vi "Sliding Menu Facade.vi"(0 "Data In":T5, 2 "Display State In":T2={"Numeric"=0.0, "Array of Button References"=[], "Space Between Menu Buttons"=0, "Number of Menu Buttons"=0, "Array of Button Names"=[], "Most Recent Vertical Position"=0, "This VI"=refnum, "Current Action"=enum."Not Moving", "Most Recent Distance Traveled"=0, "Method"=enum."Move Up", "Data In"=0}, 3 "Container State":T6) -> (6 "Data Out":T5, 7 "Display State Out":T2={"Numeric"=0.0, "Array of Button References"=[], "Space Between Menu Buttons"=0, "Number of Menu Buttons"=0, "Array of Button Names"=[], "Most Recent Vertical Position"=0, "This VI"=refnum, "Current Action"=enum."Not Moving", "Most Recent Distance Traveled"=0, "Method"=enum."Move Up", "Data In"=0}, 8 "Action":T1)   [LabVIEW 2011, in "Sliding Menu Library.lvlib" / "Sliding Menu XControl.xctl"]
uses:
  Sliding Menu XControl.xctl
  Sliding Menu Data.ctl
  <vilib>/_xctls/Container State.ctl
  Sliding Menu State.ctl
  Menu Button Library/Menu Button xControl/Menu Button xControl.xctl
  Sliding Menu SubVIs/Sliding Menu Type Definitions/Current User Action.ctl
  Sliding Menu Methods.ctl
  <vilib>/_xctls/Action.ctl
  <vilib>/_xctls/XControlSupport.lvlib
  Sliding Menu Library.lvlib
panel:
  in  "Button 7":bool(xcontrol)
  in  "Button 6":bool(xcontrol)
  in  "Button 5":bool(xcontrol)
  in  "Button 4":bool(xcontrol)
  in  "Button 3":bool(xcontrol)
  in  "Button 2":bool(xcontrol)
  in  "Button 1":bool(xcontrol)
  in  "Button 0":bool(xcontrol)
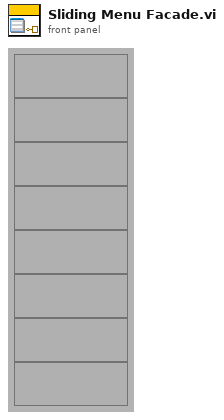
[diagram p1: front panel]
types:
  T1 = typedef "XControlSupport.lvlib/Action.ctl" = cluster{"Data Changed?":bool, "State Changed?":bool, "Action Name":string}
  T2 = typedef "Sliding Menu Library.lvlib/Sliding Menu XControl.xctl/Sliding Menu State.ctl" = cluster{"Numeric":dbl, "Array of Button References":refnum<vi>[], "Space Between Menu Buttons":i32, "Number of Menu Buttons":i32, "Array of Button Names":string[], "Most Recent Vertical Position":i32, "This VI":refnum<vi>, "Current Action":T3, "Most Recent Distance Traveled":i32, "Method":T4, "Data In":T5}
  T3 = typedef "Sliding Menu Library.lvlib/Current User Action.ctl" = enum16{"Not Moving", "Mouse Down", "Mouse Up No Dragging", "Bounce Up Needed", "Bounce Down Needed", "Dragging", "Easing"}
  T4 = typedef "Sliding Menu Methods.ctl" = enum16{"Resize", "Move Up", "Move Down", "Move to 0"}
  T5 = typedef "Sliding Menu Library.lvlib/Sliding Menu XControl.xctl/Sliding Menu Data.ctl" = i32
  T6 = typedef "XControlSupport.lvlib/Container State.ctl" = cluster{"Indicator?":bool, "Run Mode?":bool, " Refnum":refnum<vi>}
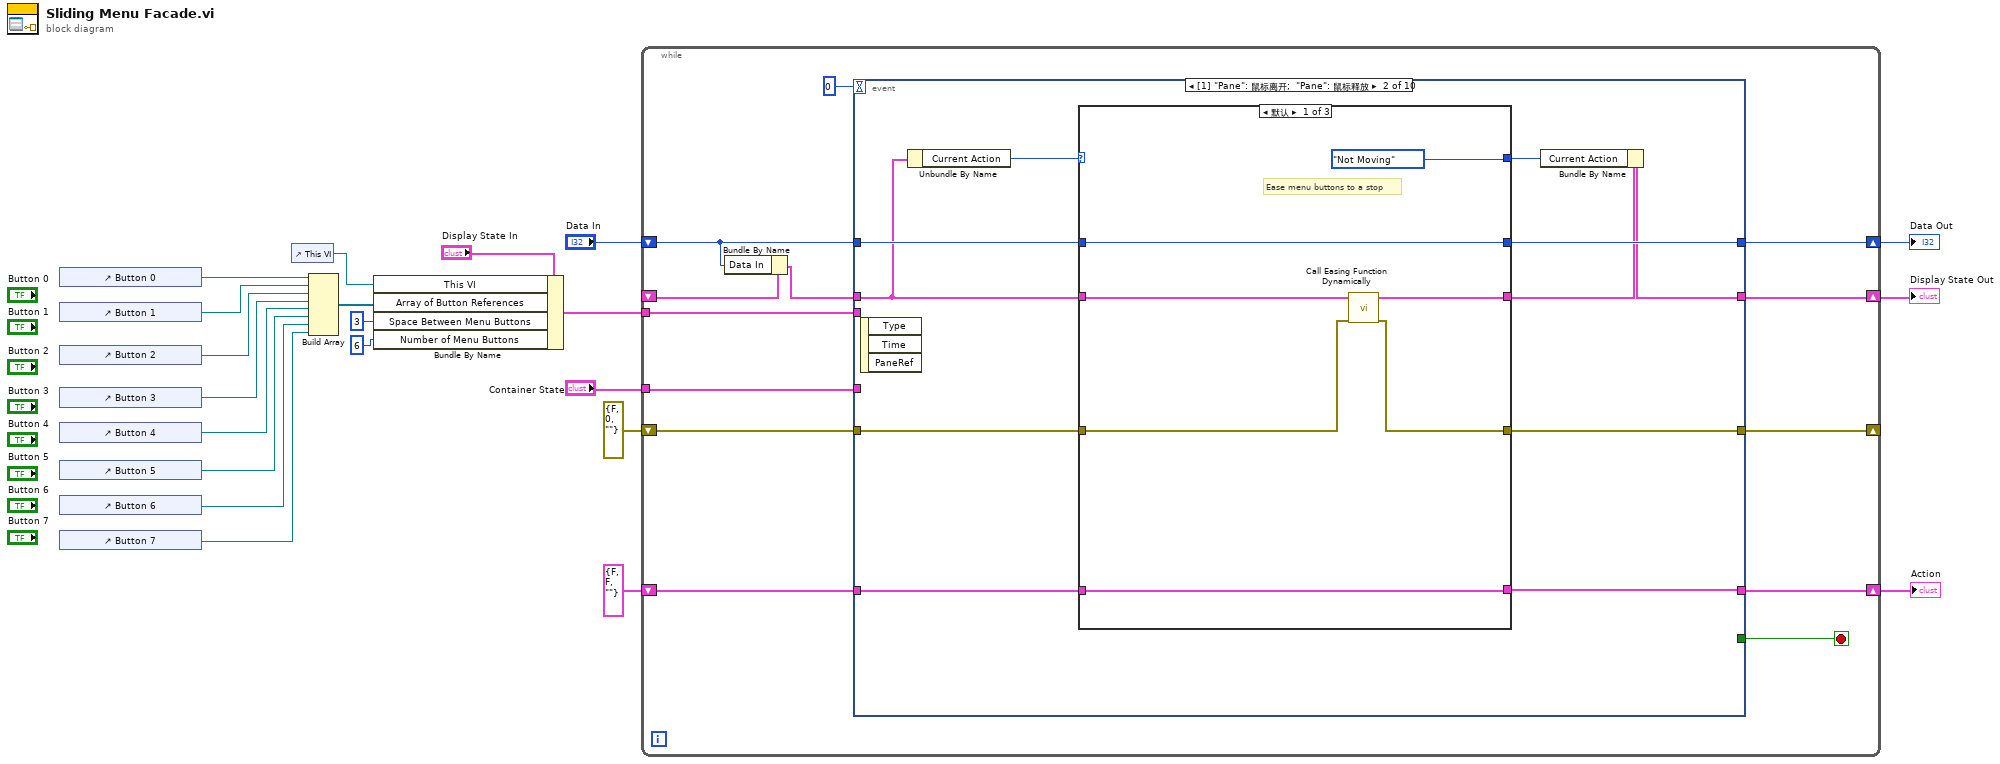
[diagram p0: block diagram]
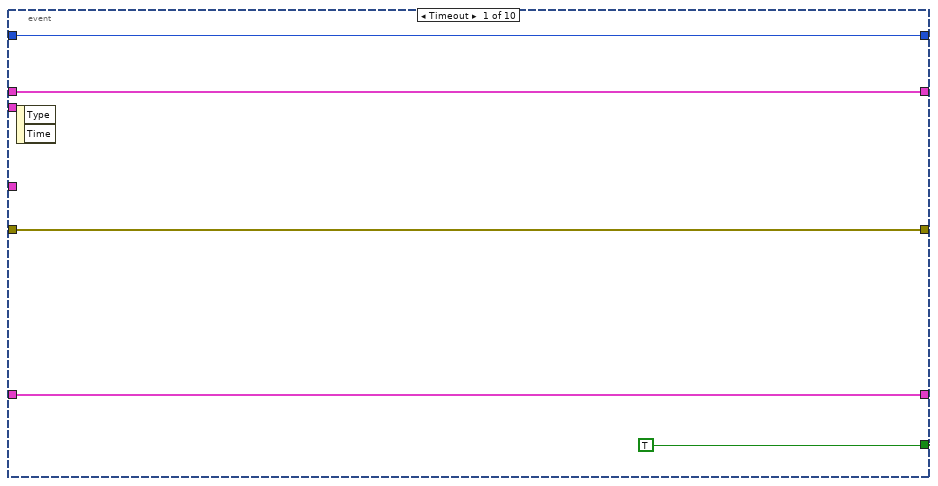
[diagram p2: hidden frame]
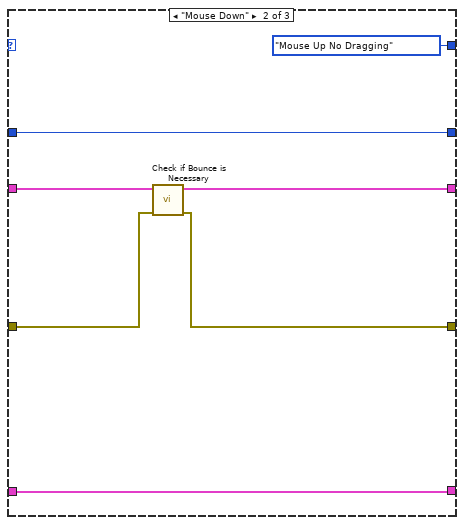
[diagram p3: hidden frame]
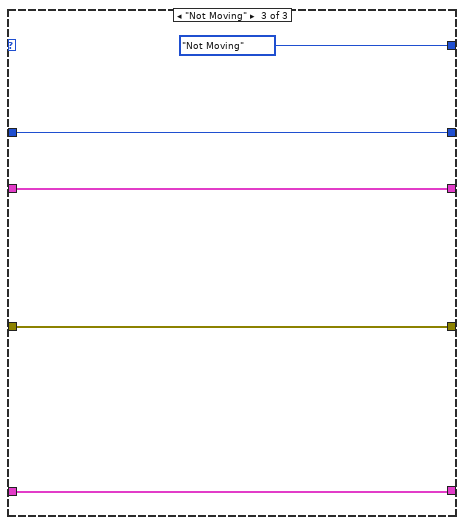
[diagram p4: hidden frame]
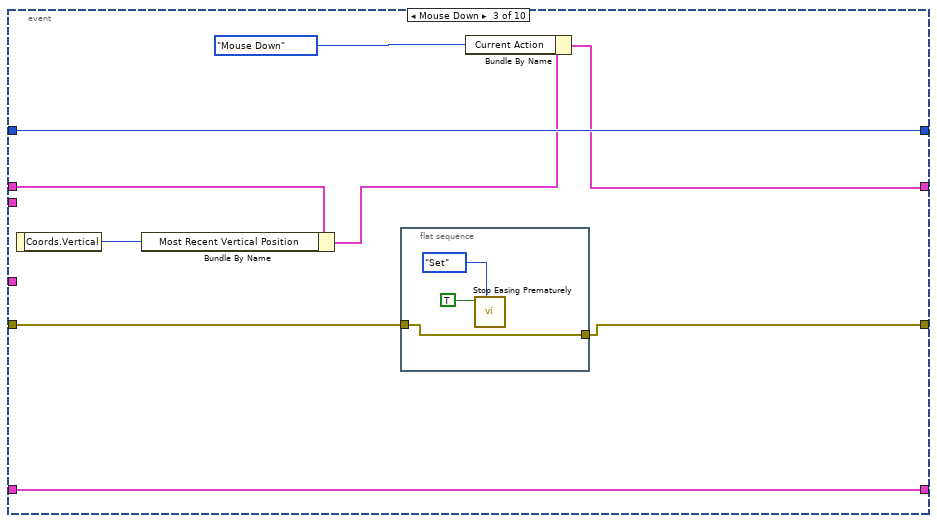
[diagram p5: hidden frame]
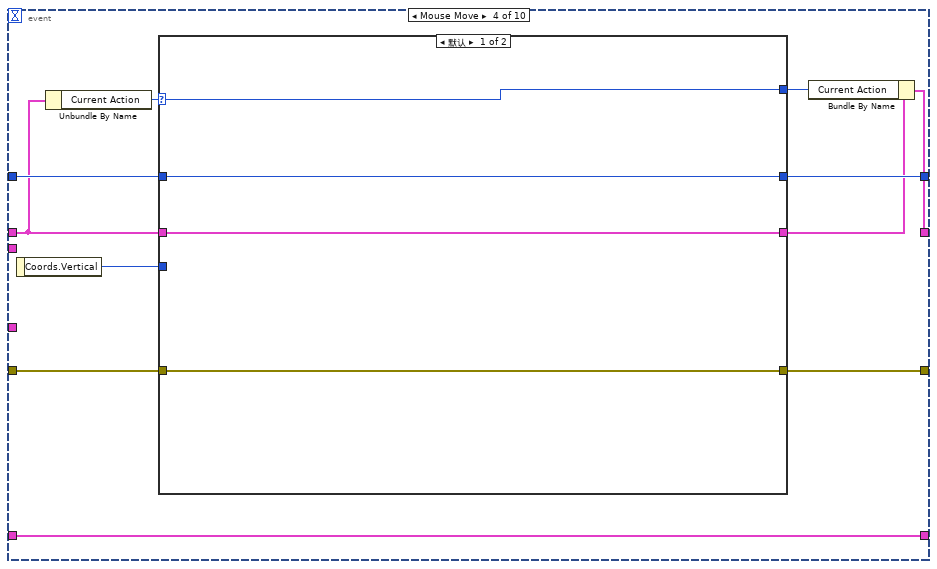
[diagram p6: hidden frame]
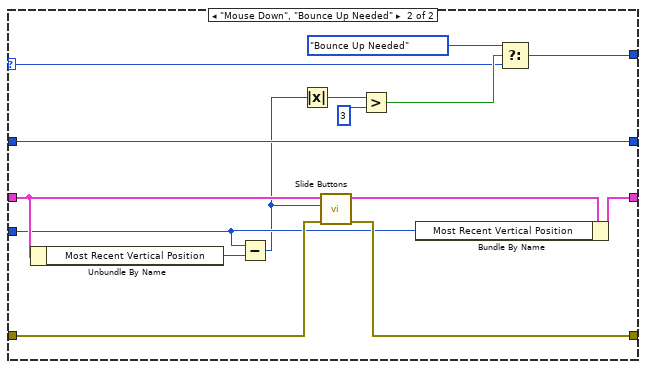
[diagram p7: hidden frame]
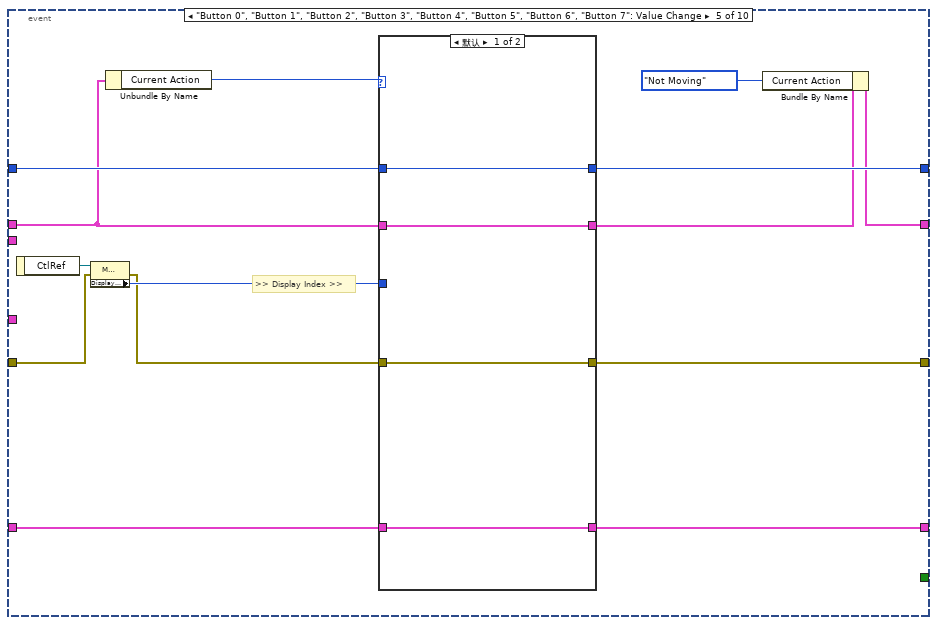
[diagram p8: hidden frame]
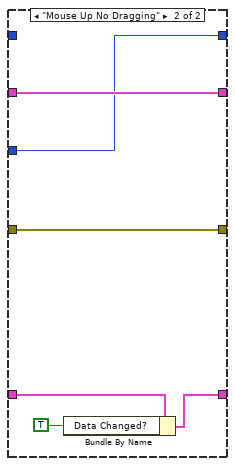
[diagram p9: hidden frame]
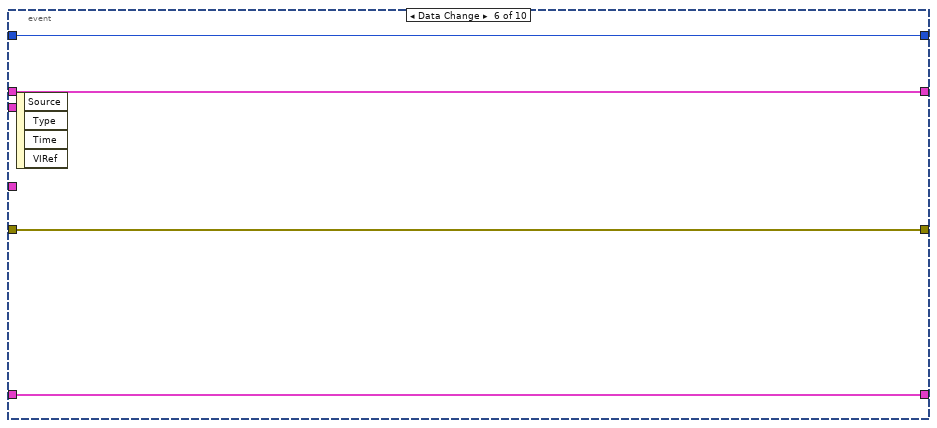
[diagram p10: hidden frame]
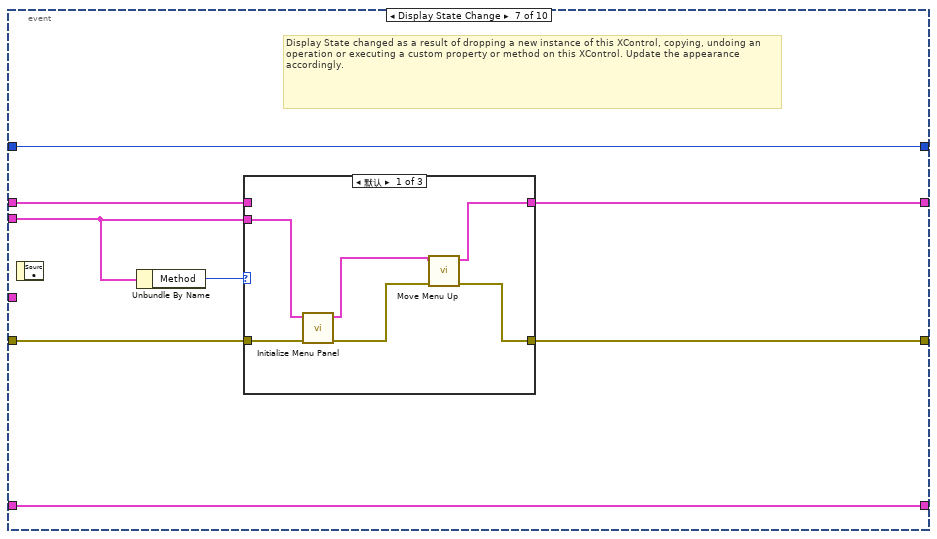
[diagram p11: hidden frame]
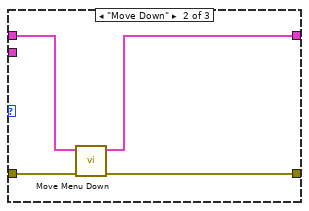
[diagram p12: hidden frame]
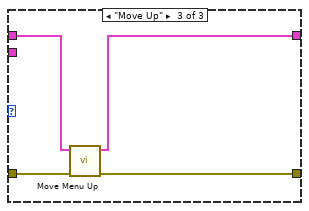
[diagram p13: hidden frame]
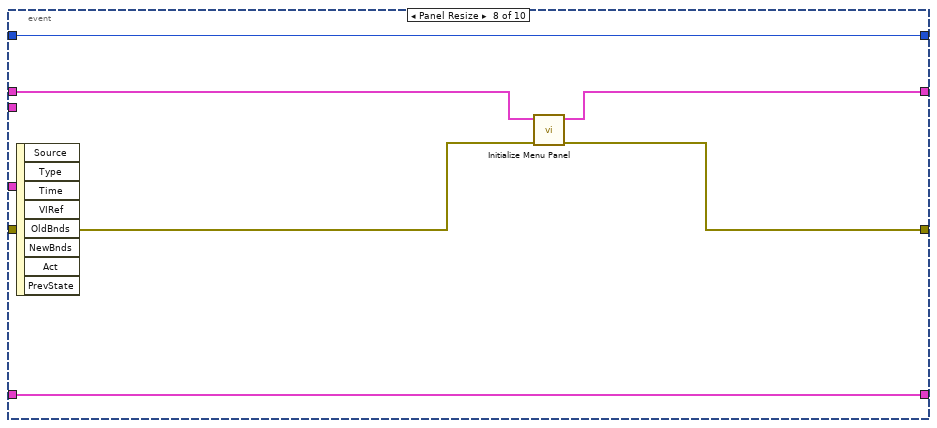
[diagram p14: hidden frame]
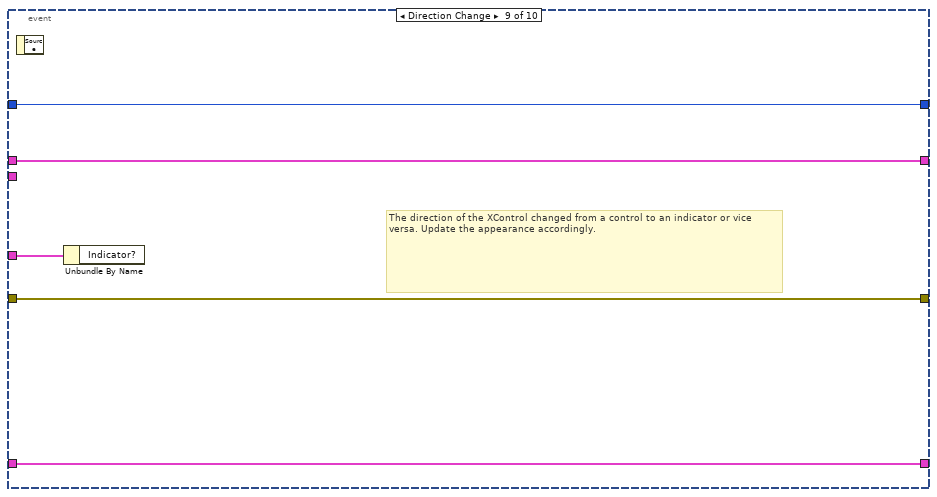
[diagram p15: hidden frame]
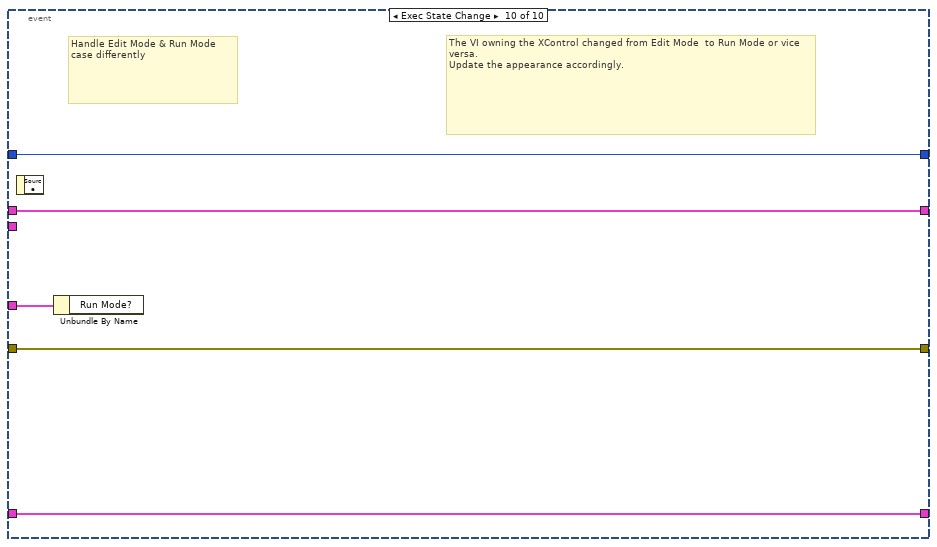
[diagram p16: hidden frame]
diagram:
  n1 = control-ref of="Button 0"() -> (w13:refnum<vi>)
  n2 = control-ref of="Button 1"() -> (w6:refnum<vi>)
  n3 = control-ref of="Button 2"() -> (w7:refnum<vi>)
  n4 = control-ref of="Button 3"() -> (w8:refnum<vi>)
  n5 = control-ref of="Button 4"() -> (w9:refnum<vi>)
  n6 = control-ref of="Button 5"() -> (w10:refnum<vi>)
  n7 = control-ref of="Button 6"() -> (w11:refnum<vi>)
  n8 = control-ref of="Button 7"() -> (w12:refnum<vi>)
  n9 = control-ref of="This VI"() -> (w4:refnum<vi>)
  n10 = Build Array(w13, w6, w7, w8, w9, w10, w11, w12) -> (w5:refnum<vi>[])
  n11 = Bundle By Name(cluster="Display State In", "This VI"=w4, "Array of Button References"=w5, "Space Between Menu Buttons"=3, "Number of Menu Buttons"=6) -> (w3:T2)
  n12 = while {
    shift-right: [w34] -> w19
    shift-left: _ -> [w25]
    tunnel: "Container State" -> [w31]
    shift-right: [w30] -> w21
    shift-left: "Data In" -> [w23]
    shift-right: [w28] -> w18
    shift-left: T1 {"Data Changed?"=FALSE, "State Changed?"=FALSE, "Action Name"=""} ("Action") -> [w29]
    shift-right: [w22] -> _
    shift-left: errorcluster {"status"=FALSE, "code"=0, "source"=""} ("error out") -> [w27]
    tunnel: w3 -> [w26]
    stop <- w33 stop-if-true
    n13 = Bundle By Name(cluster=w25, "Data In"=w23) -> (w24:T2)
    n14 = event shown="[1] \"Pane\": 鼠标离开;  \"Pane\": 鼠标释放" {
      selector: _ -> [_ _ _ _ _ _ _ _ _ _]
      dyn-events: _ -> [_ _ _ _ _ _ _ _ _ _]
      timeout: 0 -> [_ _ _ _ _ _ _ _ _ _]
      tunnel: w24 -> [w37 w45 w76 w86 w115 w138 w140 w165 w171 w176]
      tunnel: [w37 w43 w73 w83 w117 w138 w142 w164 w171 w176] -> w34
      tunnel: [TRUE _ _ _ _ _ _ _ _ _] -> w33
      tunnel: w31 -> [_ _ _ _ _ _ _ _ w172 w177]
      tunnel: w23 -> [w36 w48 w78 w90 w124 w139 w147 w167 w170 w175]
      tunnel: [w36 w49 w78 w91 w125 w139 w147 w167 w170 w175] -> w30
      tunnel: [w38 w46 w77 w92 w112 w137 w146 w166 w169 w174] -> w28
      tunnel: w29 -> [w38 w47 w77 w92 w113 w137 w146 w166 w169 w174]
      tunnel: [w35 w40 w70 w89 w123 w136 w144 w162 w168 w173] -> w22
      tunnel: w27 -> [w35 w50 w71 w88 w120 w136 w145 w163 w168 w173]
      tunnel: w26 -> [_ _ _ _ _ _ w143 _ _ _]
      event Timeout {
        n15 = event-data() -> ()  [unwired: 1 in, 2 out]
      }
      event Mouse Leave; Mouse Up {
        n16 = event-data() -> ()  [unwired: 1 in, 3 out]
        n17 = Unbundle By Name(w45) -> ("Current Action"=w41:T3)
        n18 = case shown="默认" w41 {
          tunnel: [Current_User_Action."Not Moving" ("Current Action") Current_User_Action."Mouse Up No Dragging" ("Current Action") Current_User_Action."Not Moving" ("Current Action")] -> w42
          tunnel: [w51 w58 w69] -> w40
          tunnel: w50 -> [w54 w59 w69]
          tunnel: [w56 w63 w68] -> w49
          tunnel: w48 -> [w56 w63 w68]
          tunnel: [w52 w60 w67] -> w44
          tunnel: w45 -> [w53 w61 w67]
          tunnel: [w55 w62 w66] -> w46
          tunnel: w47 -> [w55 w62 w66]
          frame Default {
            # "Ease menu buttons to a stop"
            n19 = call "Call Easing Function Dynamically.vi"("error in"=w54, "Display State In"=w53) -> ("error out"=w51:errorcluster, "Display State Out"=w52:T2)  [unwired: 8 in]
          }
          frame "Mouse Down" {
            n20 = call "Check if Bounce is Necessary.vi"("error in"=w59, "Display State In"=w61) -> ("error out"=w58:errorcluster, "Display State Out 2"=w60:T2)  [unwired: 7 in, 1 out]
          }
          frame "Not Moving" {
          }
        }
        n21 = Bundle By Name(cluster=w44, "Current Action"=w42) -> (w43:T2)
      }
      event Mouse Down {
        n22 = event-data() -> ("Coords.Vertical"=w75:i32)  [unwired: 1 in]
        n23 = Bundle By Name(cluster=w76, "Most Recent Vertical Position"=w75) -> (w72:T2)
        n24 = flat-sequence {
          tunnel: w71 -> [w79]
          tunnel: [w79] -> w70
          frame #0 {
            n25 = call "Stop Easing Prematurely.vi"("Set or Get Value"=enum16{"Set", "Get"}."Set", "Stop?"=TRUE) -> ()  [unwired: 9 in, 1 out]
          }
        }
        n26 = Bundle By Name(cluster=w72, "Current Action"=Current_User_Action."Mouse Down") -> (w73:T2)
      }
      event Mouse Move {
        n27 = event-data() -> ("Coords.Vertical"=w87:i32)  [unwired: 1 in]
        n28 = Unbundle By Name(w86) -> ("Current Action"=w85:T3)
        n29 = case shown="默认" w85 {
          selector: w85 -> [w93 w99]
          tunnel: [w93 w98] -> w82
          tunnel: [w94 w111] -> w91
          tunnel: w90 -> [w94 w111]
          tunnel: [w95 w104] -> w84
          tunnel: w86 -> [w95 w107]
          tunnel: [w96 w109] -> w89
          tunnel: w88 -> [w96 w110]
          tunnel: w87 -> [_ w106]
          frame Default {
          }
          frame "Mouse Down", "Bounce Up Needed" {
            n30 = Unbundle By Name(w107) -> ("Most Recent Vertical Position"=w108:i32)
            n31 = Subtract(x=w106, y=w108) -> (x-y=w100:i32)
            n32 = Absolute Value(x=w100) -> (abs(x)=w101:i32)
            n33 = call "Slide Buttons.vi"("error in (no error)"=w110, "Distance"=w100, "Display State In"=w107) -> ("error out"=w109:errorcluster, "Display State Out"=w105:T2)  [unwired: 7 in]
            n34 = Greater?(x=w101, y=3) -> (0:w102:bool)
            n35 = Bundle By Name(cluster=w105, "Most Recent Vertical Position"=w106) -> (w104:T2)
            n36 = Select(t=Current_User_Action."Bounce Up Needed", s=w102, f=w99) -> (s? t:f=w98:T3)
          }
        }
        n37 = Bundle By Name(cluster=w84, "Current Action"=w82) -> (w83:T2)
      }
      event "Button 0", "Button 1", "Button 2", "Button 3", "Button 4", "Button 5", "Button 6", "Button 7": Value Change {
        # ">> Display Index >>"
        n38 = event-data() -> ("CtlRef"=w122:refnum<vi>)  [unwired: 1 in]
        n39 = property class="Menu Button xControl (strict)"(reference=w122, error in=w120) -> (error out=w119:errorcluster, "Display Index"=w121:i32)  [unwired: 1 out]
        n40 = Unbundle By Name(w115) -> ("Current Action"=w114:T3)
        n41 = case shown="默认" w114 {
          tunnel: [w129 w133] -> w125
          tunnel: w124 -> [w129 _]
          tunnel: w115 -> [w128 w135]
          tunnel: [w128 w135] -> w118
          tunnel: [w127 w134] -> w123
          tunnel: w119 -> [w127 w134]
          tunnel: w121 -> [_ w133]
          tunnel: w113 -> [w126 w132]
          tunnel: [w126 w131] -> w112
          frame Default {
          }
          frame "Mouse Up No Dragging" {
            n42 = Bundle By Name(cluster=w132, "Data Changed?"=TRUE) -> (w131:T1)
          }
        }
        n43 = Bundle By Name(cluster=w118, "Current Action"=Current_User_Action."Not Moving") -> (w117:T2)
      }
      event Data Change {
        n44 = event-data() -> ()  [unwired: 1 in, 4 out]
      }
      event Display State Change {
        # "Display State changed as a result of dropping a new instance of this XControl, copying, undoing an operation or executing a custom property or method on this XControl. Update the appearance accordingly."
        n45 = event-data() -> ()  [unwired: 1 in, 1 out]
        n46 = Unbundle By Name(w143) -> ("Method"=w141:T4)
        n47 = case shown="默认" w141 {
          tunnel: w145 -> [w153 w157 w161]
          tunnel: [w148 w156 w160] -> w144
          tunnel: w143 -> [w152 _ _]
          tunnel: [w151 w154 w158] -> w142
          tunnel: w140 -> [_ w155 w159]
          frame Default {
            n48 = call "Initialize Menu Panel.vi"("error in"=w153, "Display State In"=w152) -> ("error IO 2"=w149:errorcluster, "Display State Out"=w150:T2)  [unwired: 8 in]
            n49 = call "Move Menu Up.vi"("error in (no error)"=w149, "Display State In"=w150) -> ("error out"=w148:errorcluster, "Display State Out"=w151:T2)  [unwired: 8 in]
          }
          frame "Move Down" {
            n50 = call "Move Menu Down.vi"("error in (no error)"=w157, "Display State In"=w155) -> ("error out"=w156:errorcluster, "Display State Out"=w154:T2)  [unwired: 8 in]
          }
          frame "Move Up" {
            n51 = call "Move Menu Up.vi"("error in (no error)"=w161, "Display State In"=w159) -> ("error out"=w160:errorcluster, "Display State Out"=w158:T2)  [unwired: 8 in]
          }
        }
      }
      event Panel Resize {
        n52 = event-data() -> ()  [unwired: 1 in, 8 out]
        n53 = call "Initialize Menu Panel.vi"("error in"=w163, "Display State In"=w165) -> ("error IO 2"=w162:errorcluster, "Display State Out"=w164:T2)  [unwired: 8 in]
      }
      event Direction Change {
        # "The direction of the XControl changed from a control to an indicator or vice versa. Update the appearance accordingly."
        n54 = event-data() -> ()  [unwired: 1 in, 1 out]
        n55 = Unbundle By Name(w172) -> ()  [unwired: 1 out]
      }
      event Exec State Change {
        # "The VI owning the XControl changed from Edit Mode  to Run Mode or vice versa.\nUpdate the appearance accordingly."
        # "Handle Edit Mode & Run Mode\ncase differently"
        n56 = event-data() -> ()  [unwired: 1 in, 1 out]
        n57 = Unbundle By Name(w177) -> ()  [unwired: 1 out]
      }
    }
  }
  "Display State Out" <- w19
  "Data Out" <- w21
  "Action" <- w18
